vi "PCF8575.vi"() -> ()   [LabVIEW 2016]
uses:
  <userlib>/CH341DLL/CH341DLL.lvlib
panel:
  in  "读/写":bool
  out "oReadBuffer out":u8[](array[numeric])=[69, 103] format="%x"
  out "function return":bool=TRUE
  in  "iIndex":u32
  in  "iWriteLength":u32=3
  in  "iWriteBuffer":u8[](array[numeric])=[64, 69, 103] format="%x"
  in  "iReadLength":u32=2
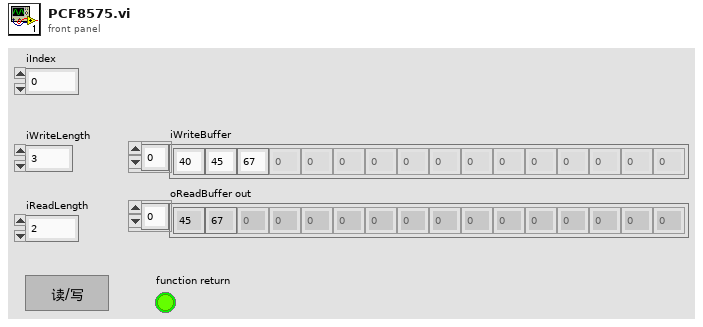
[diagram p1: front panel]
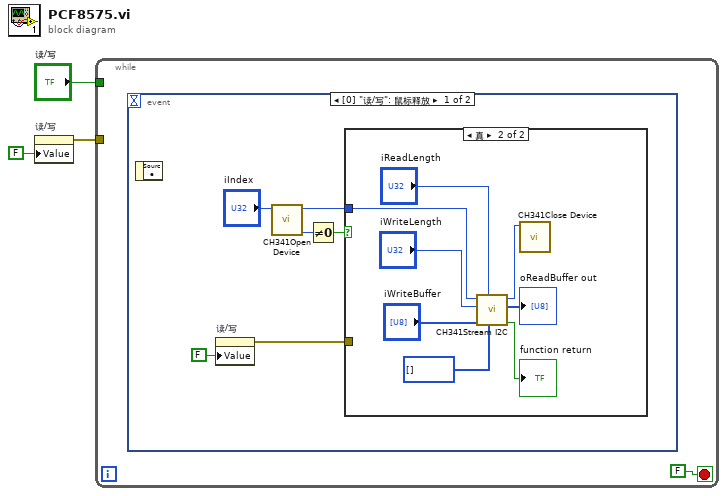
[diagram p0: block diagram]
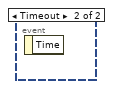
[diagram p3: hidden frame]
diagram:
  n1 = property on="读/写" class="Bool (严格)"("Value"=FALSE ("读/写I2C")) -> (error out=w3:errorcluster)  [unwired: 2 in, 1 out]
  n2 = while {
    tunnel: w3 -> [_]
    tunnel: "读/写" -> [_]
    stop <- FALSE stop-if-true
    n3 = event shown="[0] \"读/写\": 鼠标释放" {
      selector: _ -> [_ _]
      dyn-events: _ -> [_ _]
      timeout: _ -> [_ _]
      event "读/写": Mouse Up {
        n4 = event-data() -> ()  [unwired: 1 in, 1 out]
        n5 = property on="读/写" class="Bool (严格)"("Value"=FALSE ("读/写I2C")) -> (error out=w6:errorcluster)  [unwired: 2 in, 1 out]
        n6 = call <userlib>:"CH341Open Device.vi"("iIndex"="iIndex") -> ("function return"=w7:u32, "oIndex"=w9:u32)  [unwired: 8 in]
        n7 = Not Equal To 0?(x=w7) -> (x != 0?=w8:bool)
        n8 = case shown="真" w8 {
          tunnel: w9 -> [_ w12]
          tunnel: w6 -> [_ _]
          frame False {
          }
          frame True {
            n9 = call <userlib>:"CH341Stream I2C.vi"("oReadBuffer"=u8[] [], "iReadLength"="iReadLength", "iWriteBuffer"="iWriteBuffer", "iWriteLength"="iWriteLength", "iIndex"=w12) -> ("function return"=→"function return":bool, "oReadBuffer out"=→"oReadBuffer out":u32[], "oIndex"=w11:u32)  [unwired: 2 in, 1 out]
            n10 = call <userlib>:"CH341Close Device.vi"("iIndex"=w11) -> ()  [unwired: 11 in]
          }
        }
      }
      event Timeout {
        n11 = event-data() -> ()  [unwired: 1 in, 1 out]
      }
    }
  }
